vi "VISA RS485 READ new.vi"(8 "error in (no error)":errorcluster, 10 "Timeout (ms)":u32=2000, 11 "VISA resource name":refnum<visa-resource-name>="COM1") -> (0 "error out":errorcluster, 1 "Valid Read?":bool, 2 "Return String":string, 3 "dup VISA resource name":refnum<visa-resource-name>, 4 "Timeout?":bool)   [LabVIEW 2013]
doc: "VISA RS485 READ ENGINE FOR RTS"
panel:
  out "Error?":bool
  out "Corrupt Read?":bool
  # "String Read from Serial Port.  Note in\nthe Windows and Sun version the serial\nport is reset each time the VI is run, voiding\npreexisting data.  The Macintosh version\nsaves previously buffered data."
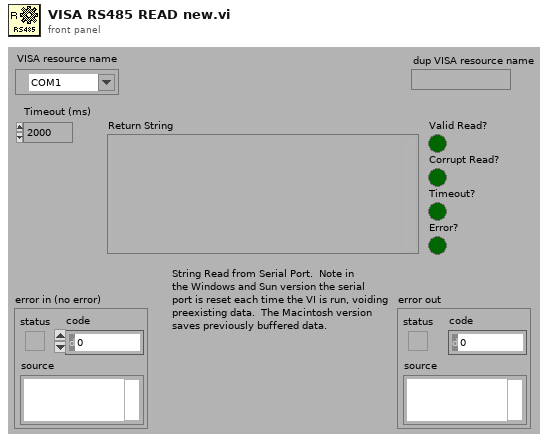
[diagram p1: front panel]
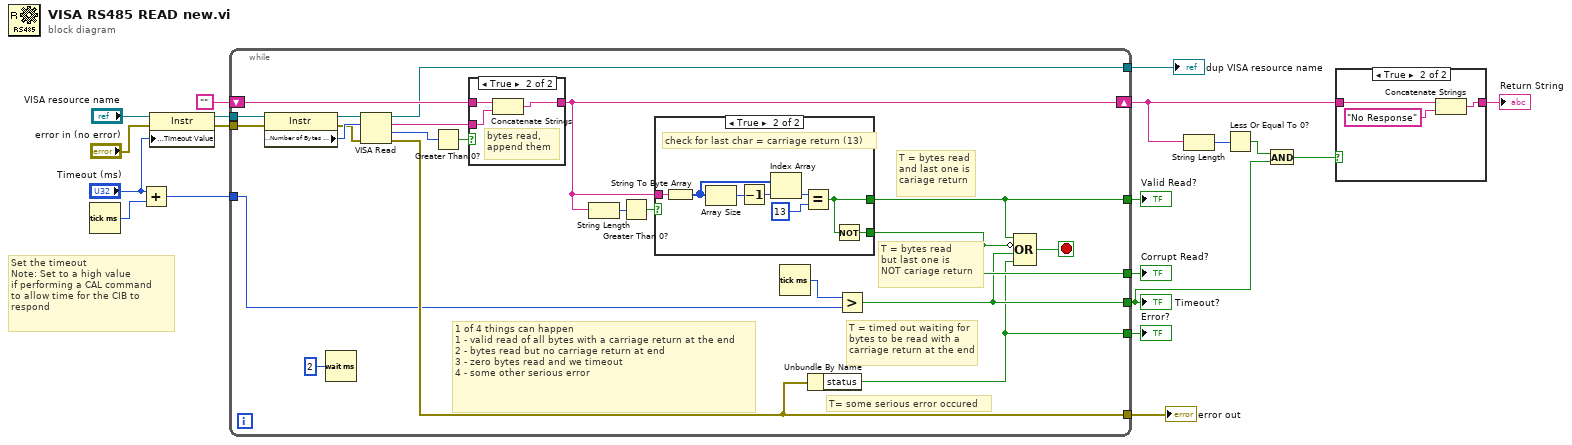
[diagram p0: block diagram]
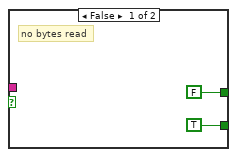
[diagram p3: hidden frame]
diagram:
  # "Set the timeout\nNote: Set to a high value\nif performing a CAL command\nto allow time for the CIB to\nrespond"
  n1 = Tick Count (ms)() -> (millisecond timer value=w15:u32)
  n2 = Add(x="Timeout (ms)", y=w15) -> (x+y=w13:u32)
  n3 = property class="Instr"(reference="VISA resource name", error in="error in (no error)", "General Settings:Timeout Value"="Timeout (ms)") -> (reference out=w16:refnum<visa-resource-name>, error out=w18:errorcluster)
  n4 = while {
    tunnel: w16 -> [w41]
    tunnel: w13 -> [w29]
    tunnel: w18 -> [w40]
    shift-right: [w31] -> w2
    shift-left: "" -> [w37]
    tunnel: [w33] -> w11
    tunnel: [w30] -> w10
    tunnel: [w26] -> w9
    tunnel: [w25] -> w4
    tunnel: [w24] -> w8
    tunnel: [w23] -> w7
    stop <- w32 stop-if-true
    # "T= some serious error occured"
    # "T = bytes read\nand last one is\ncariage return"
    # "T = bytes read\nbut last one is\nNOT cariage return"
    # "1 of 4 things can happen\n1 - valid read of all bytes with a carriage return at the end\n2 - bytes read but no carriage return at end\n3 - zero bytes read and we timeout\n4 - some other serious error"
    # "T = timed out waiting for bytes to be read with a carriage return at the end"
    n5 = property class="Instr"(reference=w41, error in=w40) -> (reference out=w22:refnum<visa-resource-name>, error out=w20:errorcluster, "Serial Settings:Number of Bytes at Serial Port"=w21:u32)
    n6 = Wait (ms)(milliseconds to wait=u32 2) -> ()  [unwired: 1 out]
    n7 = VISA Read(VISA resource name=w22, byte count=w21, error in (no error)=w20) -> (VISA resource name out=w30:refnum<visa-resource-name>, read buffer=w36:string, return count=w39:u32, error out=w33:errorcluster)
    n8 = Greater Than 0?(x=w39) -> (x > 0?=w38:bool)
    n9 = case shown="True" w38 {
      tunnel: w37 -> [w52 w55]
      tunnel: w36 -> [_ w54]
      tunnel: [w52 w53] -> w31
      frame False {
        # "no bytes read"
      }
      frame True {
        # "bytes read,\nappend them"
        n10 = Concatenate Strings(w55, w54) -> (w53:string)
      }
    }
    n11 = String Length(string=w31) -> (length=w34:i32)
    n12 = Greater Than 0?(x=w34) -> (x > 0?=w35:bool)
    n13 = case shown="True" w35 {
      tunnel: w31 -> [_ w46]
      tunnel: [FALSE w45] -> w23
      tunnel: [TRUE w44] -> w26
      frame False {
        # "no bytes read"
      }
      frame True {
        # "check for last char = carriage return (13)"
        n14 = String To Byte Array(string=w46) -> (unsigned byte array=w49:u8[])
        n15 = Array Size(array=w49) -> (size(s)=w48:i32)
        n16 = Decrement(x=w48) -> (x-1=w47:i32)
        n17 = Index Array(array=w49, index=w47) -> (element=w51:u8)
        n18 = Equal?(x=w51, y=u8 13) -> (x = y?=w45:bool)
        n19 = Not(x=w45) -> (.not. x?=w44:bool)
      }
    }
    n20 = Tick Count (ms)() -> (millisecond timer value=w28:u32)
    n21 = Unbundle By Name(w33) -> ("status"=w24:bool)
    n22 = Greater?(x=w28, y=w29) -> (0:w25:bool)
    n23 = Compound Arithmetic op=OR(w23, invert w26, w25, w24) -> (w32:bool)
  }
  "dup VISA resource name" <- w10
  "error out" <- w11
  "Corrupt Read?" <- w9
  "Timeout?" <- w4
  "Error?" <- w8
  "Valid Read?" <- w7
  n24 = String Length(string=w2) -> (length=w6:i32)
  n25 = Less Or Equal To 0?(x=w6) -> (x <= 0?=w5:bool)
  n26 = And(x=w5, y=w4) -> (x .and. y?=w3:bool)
  n27 = case shown="True" w3 {
    tunnel: w2 -> [w56 w59]
    tunnel: [w56 w58] -> w1
    frame False {
    }
    frame True {
      n28 = Concatenate Strings(w59, "No Response" ("string")) -> (w58:string)
    }
  }
  "Return String" <- w1
